vi "user.org_rid.vi"(8 "error in":errorcluster, 11 "User in":refnum<class "User.lvclass">) -> (0 "error out":errorcluster, 3 "User out":refnum<class "User.lvclass">)   [LabVIEW 2020, in "User.lvclass"]
doc: "Returns the rid of the user's organization."
uses:
  User.lvclass
  User.lvclass/User.ctl
  client.lvlib
panel:
  out "out_needed out":u32
  out "org rid":string
  in  "buf":string
  in  "cap":u32
  in  "out_needed":u32
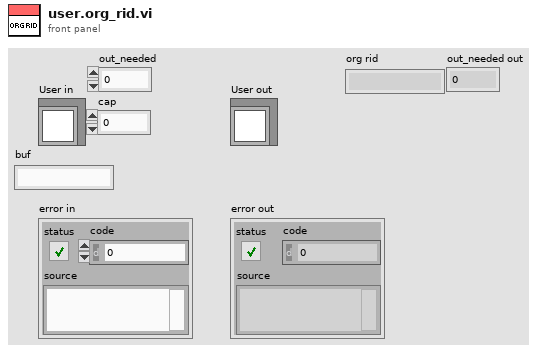
[diagram p1: front panel]
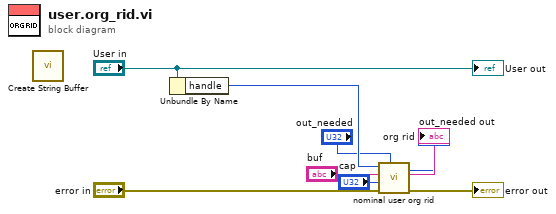
[diagram p0: block diagram]
diagram:
  n1 = call "Create String Buffer.vi"() -> ()  [unwired: 9 in, 3 out]
  n2 = Unbundle By Name("User in") -> ("handle"=w7:i32)
  n3 = call "nominal user org rid.vi"("out_needed"="out_needed", "error in (no error)"="error in", "cap"="cap", "buf"="buf", "user"=w7) -> ("error out"=→"error out":errorcluster, "buf out"=→"org rid":string, "out_needed out"=→"out_needed out":u32)  [unwired: 3 in, 1 out]
  "User out" <- "User in"
